vi "ledOnOff.vi"() -> ()   [LabVIEW 2021]
panel:
  out "LED":bool
  in  "Switch":bool
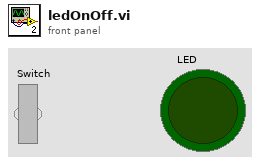
[diagram p1: front panel]
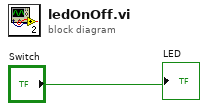
[diagram p0: block diagram]
diagram:
  "LED" <- "Switch"
